vi "Enable Disable Outuput.vi"(8 "error in (no error)":errorcluster, 10 "Enable/Disable":bool, 11 "Power Supply in":refnum<class "Power Supply.lvclass">) -> (0 "error out":errorcluster, 3 "Power Supply out":refnum<class "Power Supply.lvclass">)   [LabVIEW 2020, in "Power Supply.lvlib" / "Power Supply.lvclass"]
uses:
  Power Supply.lvclass
  Power Supply.lvclass/Power Supply.ctl
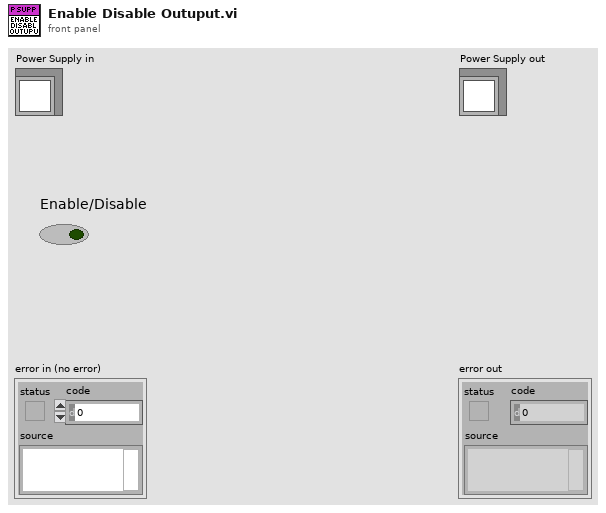
[diagram p1: front panel]
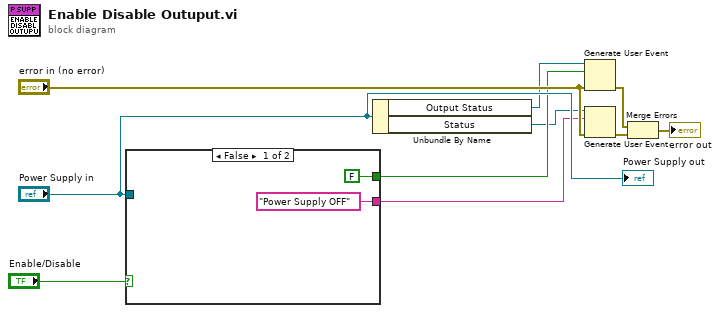
[diagram p0: block diagram]
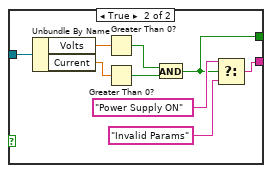
[diagram p2: hidden frame]
diagram:
  n1 = case shown="False" "Enable/Disable" {
    tunnel: "Power Supply in" -> [_ w21]
    tunnel: [FALSE w14] -> w5
    tunnel: ["Power Supply OFF" ("event data") w15] -> w3
    frame False {
    }
    frame True {
      n2 = Unbundle By Name(w21) -> ("Volts"=w19:dbl, "Current"=w20:dbl)
      n3 = Greater Than 0?(x=w19) -> (x > 0?=w18:bool)
      n4 = Greater Than 0?(x=w20) -> (x > 0?=w17:bool)
      n5 = And(x=w18, y=w17) -> (x .and. y?=w14:bool)
      n6 = Select(t="Power Supply ON" ("event data"), s=w14, f="Invalid Params" ("event data")) -> (s? t:f=w15:string)
    }
  }
  n7 = Unbundle By Name("Power Supply in") -> ("Output Status"=w6:refnum<user-event>, "Status"=w4:refnum<user-event>)
  n8 = Generate User Event(user event=w6, event data cluster=w5, error in="error in (no error)") -> (error out=w2:errorcluster)  [unwired: 1 in, 1 out]
  n9 = Generate User Event(user event=w4, event data cluster=w3, error in="error in (no error)") -> (error out=w1:errorcluster)  [unwired: 1 in, 1 out]
  n10 = Merge Errors(w2, w1) -> (→"error out":errorcluster)
  "Power Supply out" <- "Power Supply in"
